vi "ConfigurationsWindow.vi"(8 "error in (no error)":errorcluster) -> (0 "error out":errorcluster, 2 "Plik out":path, 3 "Conf":bool[](array[boolean]))   [LabVIEW 2021]
uses:
  <vilib>/Utility/miscctls.llb/LVRectTypeDef.ctl
  <vilib>/Utility/miscctls.llb/LVPoint32TypeDef.ctl
  <vilib>/Utility/miscctls.llb/LVBoundsTypeDef.ctl
panel:
  out "Coords":T1
  out "Window Bounds":T2
  out "Is Window Dragged?":bool
  in  "Tab":enum32{"Page 1"}(tab)
  in  "Plik":path
  in  "Nazwa pliku":string
  in  "Save":bool
  in  "Wartości referencyjne":string(combo)="Obliczone"
  in  "Dane przychodzące":string(combo)="Z pliku"
  out "WindowHandler":bool=TRUE
  out "Komunikat":string caption="Wpisz kod"
  in  "Stop":bool
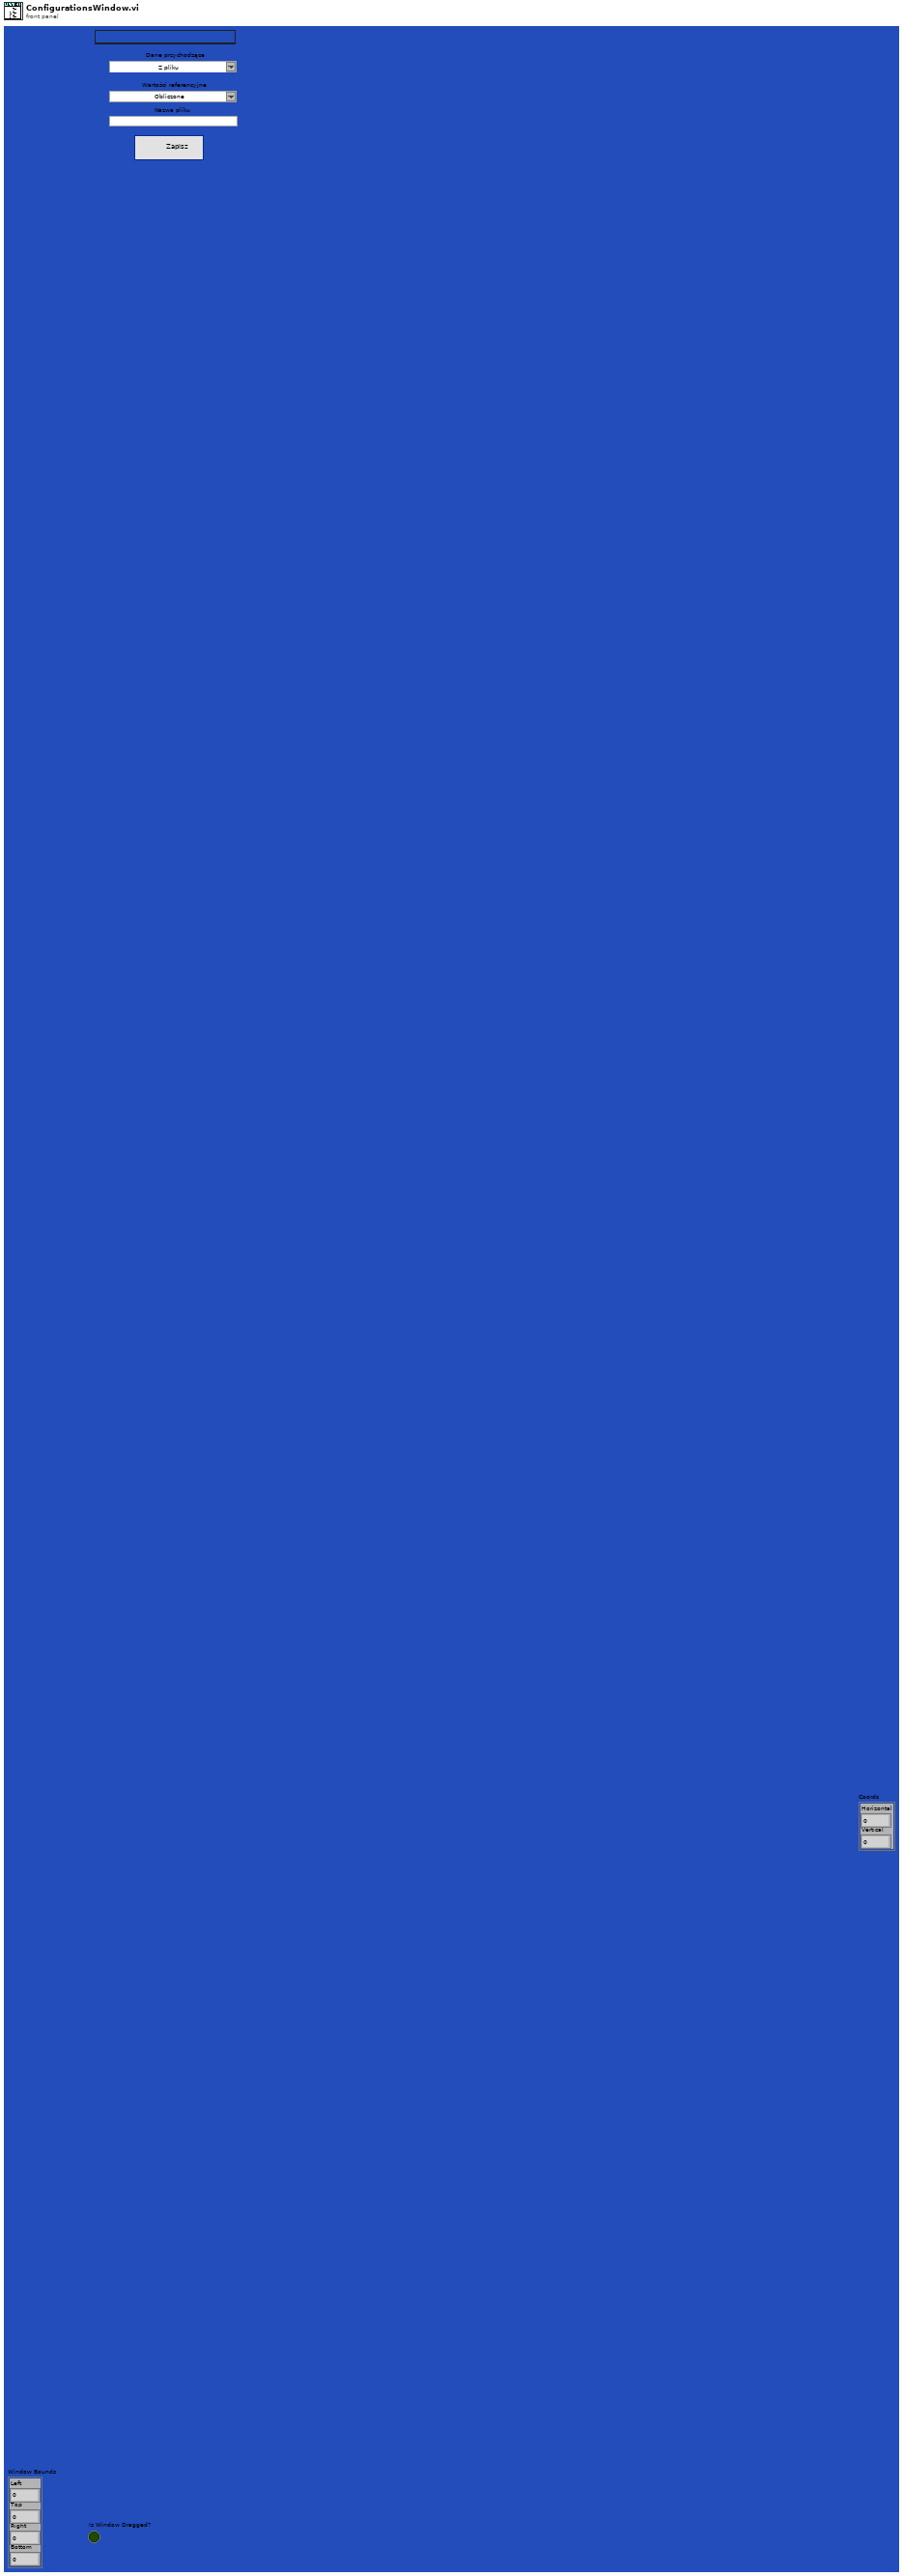
[diagram p1: front panel]
types:
  T1 = typedef "LVPoint32TypeDef.ctl" = cluster{"Horizontal":i32, "Vertical":i32}
  T2 = typedef "LVRectTypeDef.ctl" = cluster{"Left":i16, "Top":i16, "Right":i16, "Bottom":i16}
  T3 = typedef "LVBoundsTypeDef.ctl" = cluster{"Width":u32, "Height":u32}
  T4 = cluster{"Horizontal":i16, "Vertical":i16, "Horizontal":i16, "Vertical":i16}
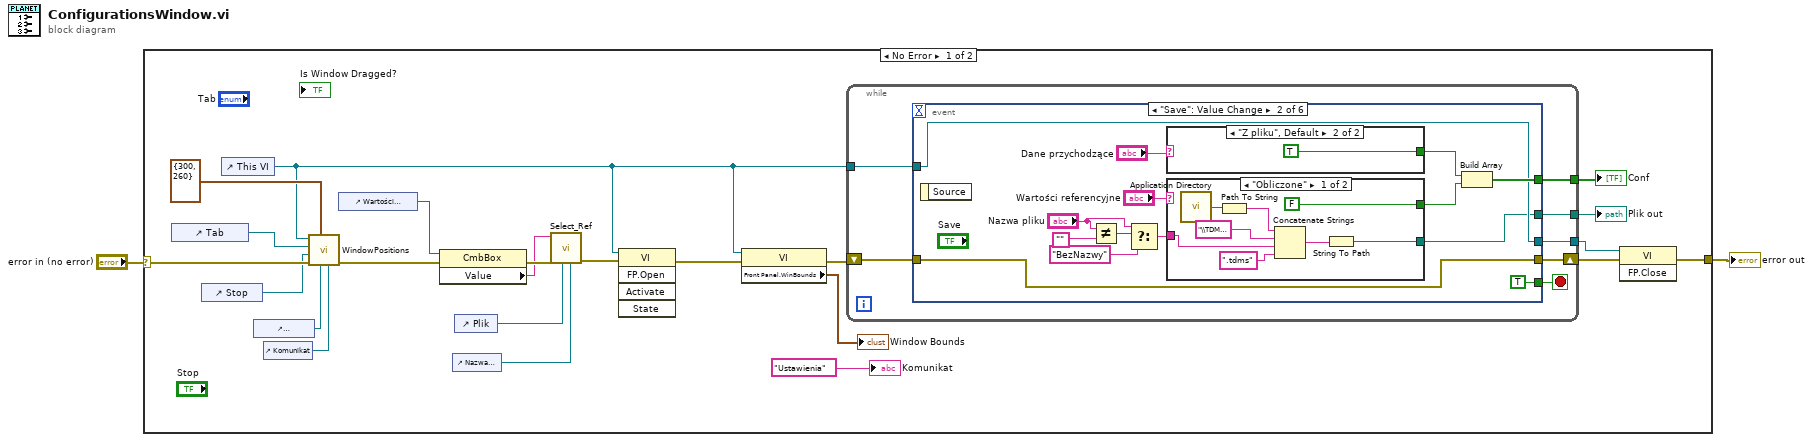
[diagram p0: block diagram]
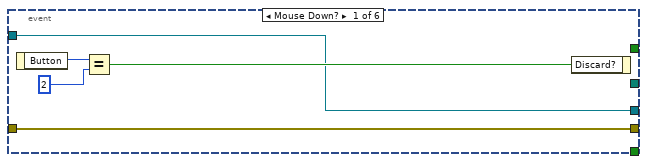
[diagram p2: hidden frame]
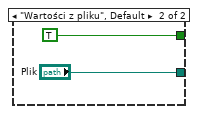
[diagram p3: hidden frame]
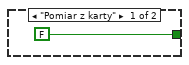
[diagram p4: hidden frame]
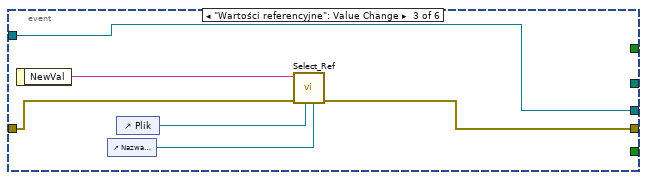
[diagram p5: hidden frame]
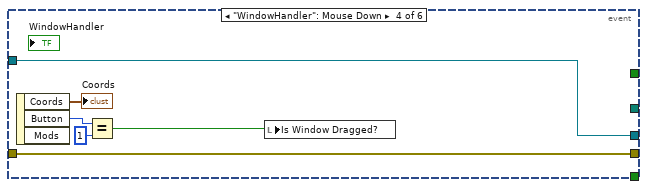
[diagram p6: hidden frame]
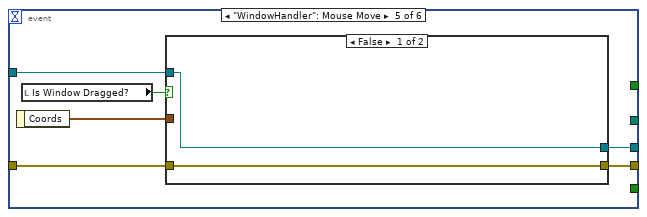
[diagram p7: hidden frame]
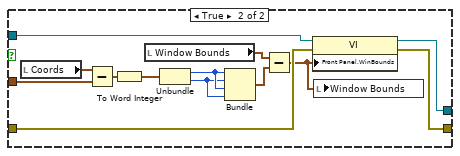
[diagram p8: hidden frame]
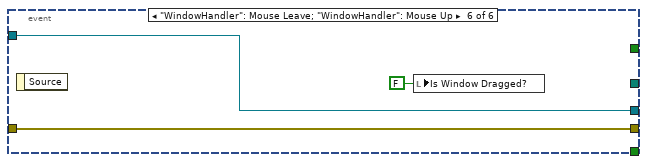
[diagram p9: hidden frame]
diagram:
  n1 = case shown="No Error" "error in (no error)" {
    selector: "error in (no error)" -> [w13 w100]
    tunnel: [w17 w100] -> w2
    frame No Error {
      n2 = control-ref of="Tab"() -> (w22:refnum<vi>)
      n3 = control-ref of="Stop"() -> (w12:refnum<vi>)
      n4 = control-ref of="This VI"() -> (w3:refnum<vi>)
      n5 = control-ref of="WindowHandler"() -> (w21:refnum<vi>)
      n6 = control-ref of="Komunikat"() -> (w20:refnum<vi>)
      n7 = call "WindowPositions.vi"("Komunikat"=w20, "WindowHandler"=w21, "Dim"=T3 {"Width"=300, "Height"=260} ("Tab Control Pane Dimension"), "error in (no error)"=w13, "Stop"=w12, "Tab"=w22, "VI in"=w3) -> ("error out"=w11:errorcluster)  [unwired: 4 in]
      n8 = control-ref of="Wartości referencyjne"() -> (w10:refnum<vi>)
      n9 = property class="CmbBox"(reference=w10, error in=w11) -> (error out=w9:errorcluster, "Value"=w8:string)  [unwired: 1 out]
      n10 = control-ref of="Nazwa pliku"() -> (w7:refnum<vi>)
      n11 = control-ref of="Plik"() -> (w6:refnum<vi>)
      n12 = call "Select_Ref.vi"("Nazwa pliku"=w7, "Path in"=w6, "error in (no error)"=w9, "NewVal"=w8) -> ("error out"=w5:errorcluster)  [unwired: 7 in]
      n13 = invoke class="VI" method="FP.Open"(reference=w3, error in=w5) -> (error out=w4:errorcluster)  [unwired: 3 in, 4 out]
      n14 = property class="VI"(reference=w3, error in=w4) -> (error out=w25:errorcluster, "Front Panel.WinBounds"=→"Window Bounds":T2)  [unwired: 1 out]
      n15 = while {
        shift-right: [w30] -> w18
        shift-left: w25 -> [w32]
        tunnel: w3 -> [w29]
        tunnel: [w28] -> w16
        tunnel: [w27] -> w15
        tunnel: [w26] -> w14
        stop <- w31 stop-if-true
        n16 = event shown="[1] \"Save\": Value Change" {
          selector: _ -> [_ _ _ _ _ _]
          dyn-events: _ -> [_ _ _ _ _ _]
          timeout: _ -> [_ _ _ _ _ _]
          tunnel: w32 -> [w34 w51 w69 w71 w79 w98]
          tunnel: [w34 w51 w68 w71 w78 w98] -> w30
          tunnel: [_ TRUE _ _ _ _] -> w31
          tunnel: w29 -> [w33 w46 w67 w70 w77 w97]
          tunnel: [_ w47 _ _ _ _] -> w28
          tunnel: [w33 w46 w67 w70 w76 w97] -> w27
          tunnel: [_ w43 _ _ _ _] -> w26
          event Mouse Down? {
            n17 = event-data() -> ("Button"=w37:u16)  [unwired: 1 in]
            n18 = Equal?(x=w37, y=u16 2) -> (x = y?=w35:bool)
            n19 = event-data("Discard?"=w35) -> ()  [unwired: 1 in, 1 out]
          }
          event "Save": Value Change {
            n20 = event-data() -> ()  [unwired: 1 in, 1 out]
            n21 = Not Equal?(x="Nazwa pliku", y="") -> (x != y?=w41:bool)
            n22 = Select(t="Nazwa pliku", s=w41, f="BezNazwy") -> (s? t:f=w38:string)
            n23 = case shown="\"Z pliku\", Default" "Dane przychodzące" {
              tunnel: [FALSE TRUE] -> w49
              frame "Pomiar z karty" {
              }
              frame "Z pliku", Default {
              }
            }
            n24 = case shown="\"Obliczone\"" "Wartości referencyjne" {
              tunnel: [FALSE TRUE] -> w48
              tunnel: [w53 "Plik"] -> w43
              tunnel: w38 -> [w52 _]
              frame "Obliczone" {
                n25 = call <vilib>:"Application Directory.vi"() -> ("Application Directory"=w56:path)
                n26 = Path To String(path=w56) -> (string=w57:string)
                n27 = Concatenate Strings(w57, "\\TDMS_Save\\" ("string"), w52, ".tdms" ("string")) -> (w58:string)
                n28 = String To Path(string=w58) -> (path=w53:path)
              }
              frame "Wartości z pliku", Default {
              }
            }
            n29 = Build Array(w49, w48) -> (w47:bool[])
          }
          event "Wartości referencyjne": Value Change {
            n30 = event-data() -> ("NewVal"=w66:string)  [unwired: 1 in]
            n31 = control-ref of="Nazwa pliku"() -> (w64:refnum<vi>)
            n32 = control-ref of="Plik"() -> (w65:refnum<vi>)
            n33 = call "Select_Ref.vi"("Nazwa pliku"=w64, "Path in"=w65, "error in (no error)"=w69, "NewVal"=w66) -> ("error out"=w68:errorcluster)  [unwired: 7 in]
          }
          event "WindowHandler": Mouse Down {
            n34 = event-data() -> ("Coords"=→"Coords":T1, "Button"=w74:u16)  [unwired: 1 in, 1 out]
            n35 = Equal?(x=w74, y=u16 1) -> (x = y?=w72:bool)
            n36 = local write "Is Window Dragged?"(w72) -> ()
          }
          event "WindowHandler": Mouse Move {
            n37 = event-data() -> ("Coords"=w80:T1)  [unwired: 1 in]
            n38 = local read "Is Window Dragged?"() -> (w81:bool)
            n39 = case shown="False" w81 {
              tunnel: w80 -> [_ w91]
              tunnel: w79 -> [w83 w88]
              tunnel: [w83 w87] -> w78
              tunnel: w77 -> [w82 w85]
              tunnel: [w82 w84] -> w76
              frame False {
              }
              frame True {
                n40 = local read "Coords"() -> (w92:T1)
                n41 = Subtract(x=w92, y=w91) -> (x-y=w96:T1)
                n42 = To Word Integer(number=w96) -> (16bit integer=w95:cluster{"Horizontal":i16, "Vertical":i16})
                n43 = local read "Window Bounds"() -> (w90:T2)
                n44 = Unbundle(w95) -> ("Horizontal"=w94:i16, "Vertical"=w93:i16)
                n45 = Bundle("Horizontal"=w94, "Vertical"=w93, "Horizontal"=w94, "Vertical"=w93) -> (w89:T4)  [unwired: 1 in]
                n46 = Subtract(x=w90, y=w89) -> (x-y=w86:T2)
                n47 = property class="VI"(reference=w85, error in=w88, "Front Panel.WinBounds"=w86) -> (reference out=w84:refnum<vi>, error out=w87:errorcluster)
                n48 = local write "Window Bounds"(w86) -> ()
              }
            }
          }
          event "WindowHandler": Mouse Leave; "WindowHandler": Mouse Up {
            n49 = event-data() -> ()  [unwired: 1 in, 1 out]
            n50 = local write "Is Window Dragged?"(FALSE ("Is Window Dragged?")) -> ()
          }
        }
      }
      "Conf" <- w16
      "Plik out" <- w14
      n51 = invoke class="VI" method="FP.Close"(reference=w15, error in=w18) -> (error out=w17:errorcluster)  [unwired: 1 in, 2 out]
      "Komunikat" <- "Ustawienia" ("Komunikat")
    }
    frame Error {
    }
  }
  "error out" <- w2
